vi "AcknowledgeMessage.vi"(8 "error in (no error)":errorcluster, 9 "acknowledge":bool=TRUE, 10 "message header":T1, 11 "service in":refnum<class "IcmMessageService.lvclass">) -> (0 "error out":errorcluster, 3 "service out":refnum<class "IcmMessageService.lvclass">)   [LabVIEW 2017, in "IcmMessageService.lvclass"]
doc: "Sets a property on a message that indicates whether the current service acknowledges that message."
uses:
  <vilib>/addons/InsightCM/MessageBus/MessageService/IcmMessageService.lvclass
  <vilib>/addons/InsightCM/MessageBus/Base/controls/MessageHeader.ctl
  <vilib>/addons/InsightCM/MessageBus/Base/controls/KeyValuePair.ctl
  <vilib>/addons/InsightCM/MessageBus/MessageService/IcmMessageService.lvclass/IcmMessageService.ctl
  C:/Program Files (x86)/National Instruments/LabVIEW 2017/vi.lib/addons/InsightCM/Binaries/LabviewMessageAdapter.dll
  Binaries/LabviewMessageAdapter.dll
  <vilib>/addons/InsightCM/Utilities/PropertyHelpers/PropertyHelpers.lvlib
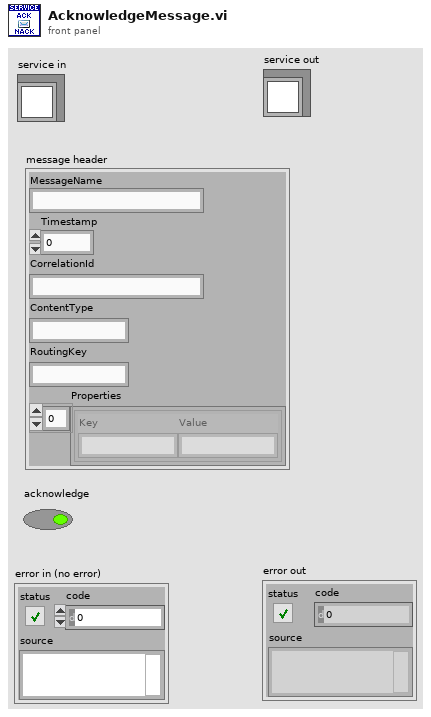
[diagram p1: front panel]
types:
  T1 = typedef "MessageHeader.ctl" = cluster{"MessageName":string, "Timestamp":i64, "CorrelationId":string, "ContentType":string, "RoutingKey":string, "Properties":T2[]}
  T2 = typedef "KeyValuePair.ctl" = cluster{"Key":string, "Value":string}
  T3 = typedef "MessageServiceDvr.ctl" = refnum<data-value>
  T4 = typedef "MessageServiceData.ctl" = cluster{"Service":refnum<k24>}
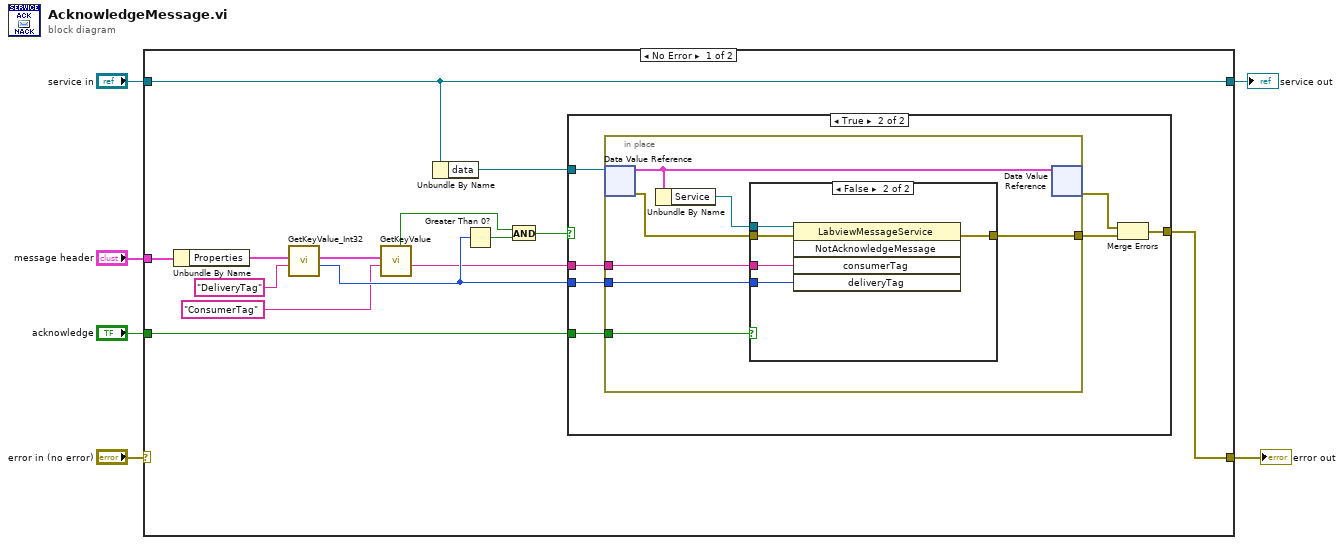
[diagram p0: block diagram]
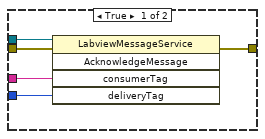
[diagram p3: hidden frame]
diagram:
  n1 = case shown="No Error" "error in (no error)" {
    selector: "error in (no error)" -> [_ w46]
    tunnel: [w19 w46] -> w1
    tunnel: "service in" -> [w14 w45]
    tunnel: [w14 w45] -> w2
    tunnel: "acknowledge" -> [w18 _]
    tunnel: "message header" -> [w17 _]
    frame No Error {
      n2 = Unbundle By Name(w17) -> ("Properties"=w13:T2[])
      n3 = call <vilib>:"GetKeyValue_Int32.vi"("key"="DeliveryTag" ("Key"), "key value pairs"=w13) -> ("value"=w10:i32, "key value pairs out"=w12:T2[])  [unwired: 7 in, 1 out]
      n4 = call <vilib>:"GetKeyValue.vi"("key"="ConsumerTag" ("Key"), "key value pairs"=w12) -> ("value"=w8:string, "found"=w7:bool)  [unwired: 7 in, 1 out]
      n5 = Unbundle By Name(w14) -> ("data"=w20:T3)
      n6 = Greater Than 0?(x=w10) -> (x > 0?=w16:bool)
      n7 = And(x=w7, y=w16) -> (x .and. y?=w15:bool)
      n8 = case shown="True" w15 {
        tunnel: w20 -> [_ w27]
        tunnel: w8 -> [_ w24]
        tunnel: [_ w23] -> w19
        tunnel: w18 -> [_ w22]
        tunnel: w10 -> [_ w21]
        frame False {
        }
        frame True {
          n9 = in-place {
            in-place-border: [w33] -> w25
            in-place-border: w24 -> [w32]
            in-place-border: w22 -> [w30]
            in-place-border: w21 -> [w31]
            n10 = in-place-dvr #1(w27) -> (w34:T4, w28:errorcluster)
            n11 = Unbundle By Name(w34) -> ("Service"=w29:refnum<k24>)
            n12 = case shown="False" w30 {
              tunnel: [w39 w44] -> w33
              tunnel: w28 -> [w38 w43]
              tunnel: w29 -> [w37 w42]
              tunnel: w32 -> [w36 w41]
              tunnel: w31 -> [w35 w40]
              frame True {
                n13 = invoke class="LabviewMessageService" method="AcknowledgeMessage"(reference=w37, error in=w38, "consumerTag"=w36, "deliveryTag"=w35) -> (error out=w39:errorcluster)  [unwired: 1 in, 4 out]
              }
              frame False {
                n14 = invoke class="LabviewMessageService" method="NotAcknowledgeMessage"(reference=w42, error in=w43, "consumerTag"=w41, "deliveryTag"=w40) -> (error out=w44:errorcluster)  [unwired: 1 in, 4 out]
              }
            }
            n15 = in-place-dvr #1(w34) -> (w26:errorcluster)  [unwired: 1 out]
          }
          n16 = Merge Errors(w26, w25) -> (w23:errorcluster)
        }
      }
    }
    frame Error {
    }
  }
  "service out" <- w2
  "error out" <- w1
